vi "21414111邱致綸.vi"() -> ()   [LabVIEW 2017]
panel:
  out "Numeric 2":dbl
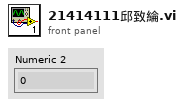
[diagram p1: front panel]
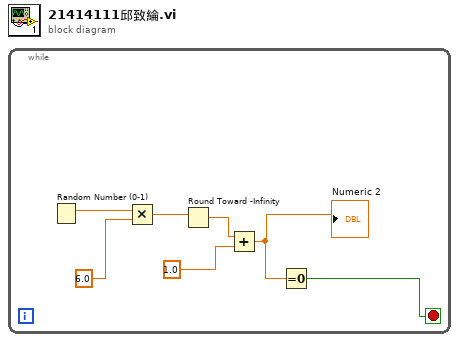
[diagram p0: block diagram]
diagram:
  n1 = while {
    stop <- w1 stop-if-true
    n2 = Random Number (0-1)() -> (number: 0 to 1=w7:dbl)
    n3 = Multiply(x=w7, y=6.0) -> (x*y=w3:dbl)
    n4 = Round Toward -Infinity(1:w3) -> (0:w4:dbl)
    n5 = Add(x=w4, y=1.0) -> (x+y=w2:dbl)
    "Numeric 2" <- w2
    n6 = Equal To 0?(x=w2) -> (x = 0?=w1:bool)
  }
